vi "DMM Configuration - Update DMM Temp Controls.vi"(8 "error in (no error)":errorcluster, 9 "DMM Temp - Value":T1={"DMM Temp - Transducer Type"=1, "DMM Temp - Thermocouple Type"=6, "DMM Temp - Fixed Reference Junction"=25.0, "DMM Temp - RTD Type"=enum."Pt3851", "DMM Temp - RTD Resistance"=100.0, "DMM Temp - Thermistor Type"=enum."44006", "DMM Temp - RTD A"=0.0039083, "DMM Temp - RTD B"=-5.775e-07, "DMM Temp - RTD C"=-4.183e-12, "DMM Temp - Thermistor A"=0.0010295, "DMM Temp - Thermistor B"=0.0002391, "DMM Temp - Thermistor C"=1.568e-07} {"DMM Temp - Thermistor C" format="%#_13g"; "DMM Temp - Thermistor B" format="%#_13g"; "DMM Temp - Thermistor A" format="%#_13g"; "DMM Temp - RTD Resistance" format="%.2f"; "DMM Temp - Fixed Reference Junction" format="%.2f"; "DMM Temp - Thermocouple Type" items=["B"=1, "E"=4, "J"=6, "K"=7, "N"=8, "R"=9, "S"=10, "T"=11]; "DMM Temp - Transducer Type" items=["Thermocouple"=1, "Thermistor"=2, "2-Wire RTD"=3, "4-Wire RTD"=4]}, 11 "Measurement Controls Refs":T6) -> (0 "error out":errorcluster)   [LabVIEW 2016, in "DMM-SWITCH-ScanList System Explorer.lvlib"]
uses:
  DMM-SWITCH-ScanList System Explorer.lvlib
  <instrlib>/niDMM/nidmm.llb/niDMM Transducer Type.ctl
  <instrlib>/niDMM/nidmm.llb/niDMM Thermistor Type.ctl
  <instrlib>/niDMM/nidmm.llb/niDMM RTD Type.ctl
  <instrlib>/niDMM/nidmm.llb/niDMM Thermocouple Type.ctl
  Configuration Controls/DMM Temp.ctl
panel:
  in  "DMM Temp - Thermocouple Type":T3=6 caption="DMM Temp - Thermocouple Type Value" items=["B"=1, "E"=4, "J"=6, "K"=7, "N"=8, "R"=9, "S"=10, "T"=11]
  in  "DMM Temp - RTD Type":T4=enum."Pt3851" caption="DMM Temp - RTD Type Value"
  in  "DMM Temp - Thermistor Type":T5=enum."44006" caption="DMM Temp - Thermistor Type Value"
  in  "DMM Temp - Transducer Type":T2=1 items=["Thermocouple"=1, "Thermistor"=2, "2-Wire RTD"=3, "4-Wire RTD"=4]
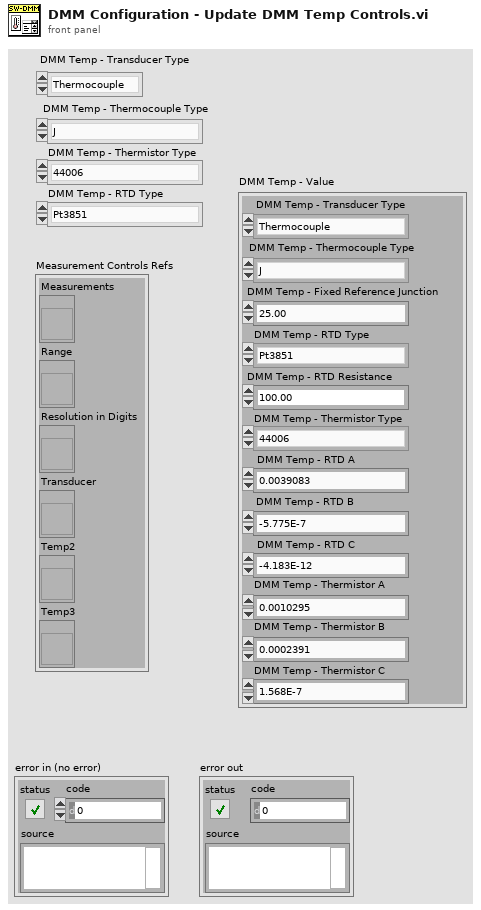
[diagram p1: front panel]
types:
  T1 = typedef "DMM-SWITCH-ScanList System Explorer.lvlib/DMM Temp.ctl" = cluster{"DMM Temp - Transducer Type":T2, "DMM Temp - Thermocouple Type":T3, "DMM Temp - Fixed Reference Junction":dbl, "DMM Temp - RTD Type":T4, "DMM Temp - RTD Resistance":dbl, "DMM Temp - Thermistor Type":T5, "DMM Temp - RTD A":dbl, "DMM Temp - RTD B":dbl, "DMM Temp - RTD C":dbl, "DMM Temp - Thermistor A":dbl, "DMM Temp - Thermistor B":dbl, "DMM Temp - Thermistor C":dbl}
  T2 = typedef "niDMM Transducer Type.ctl" = i32
  T3 = typedef "niDMM Thermocouple Type.ctl" = i32
  T4 = typedef "niDMM RTD Type.ctl" = enum16{"Custom", "Pt3750", "Pt3851", "Pt3911", "Pt3916", "Pt3920", "Pt3928"}
  T5 = typedef "niDMM Thermistor Type.ctl" = enum16{"Custom", "44004", "44006", "44007"}
  T6 = cluster{"Measurements":refnum<vi>, "Range":refnum<vi>, "Resolution in Digits":refnum<vi>, "Transducer":refnum<vi>, "Temp2":refnum<vi>, "Temp3":refnum<vi>}
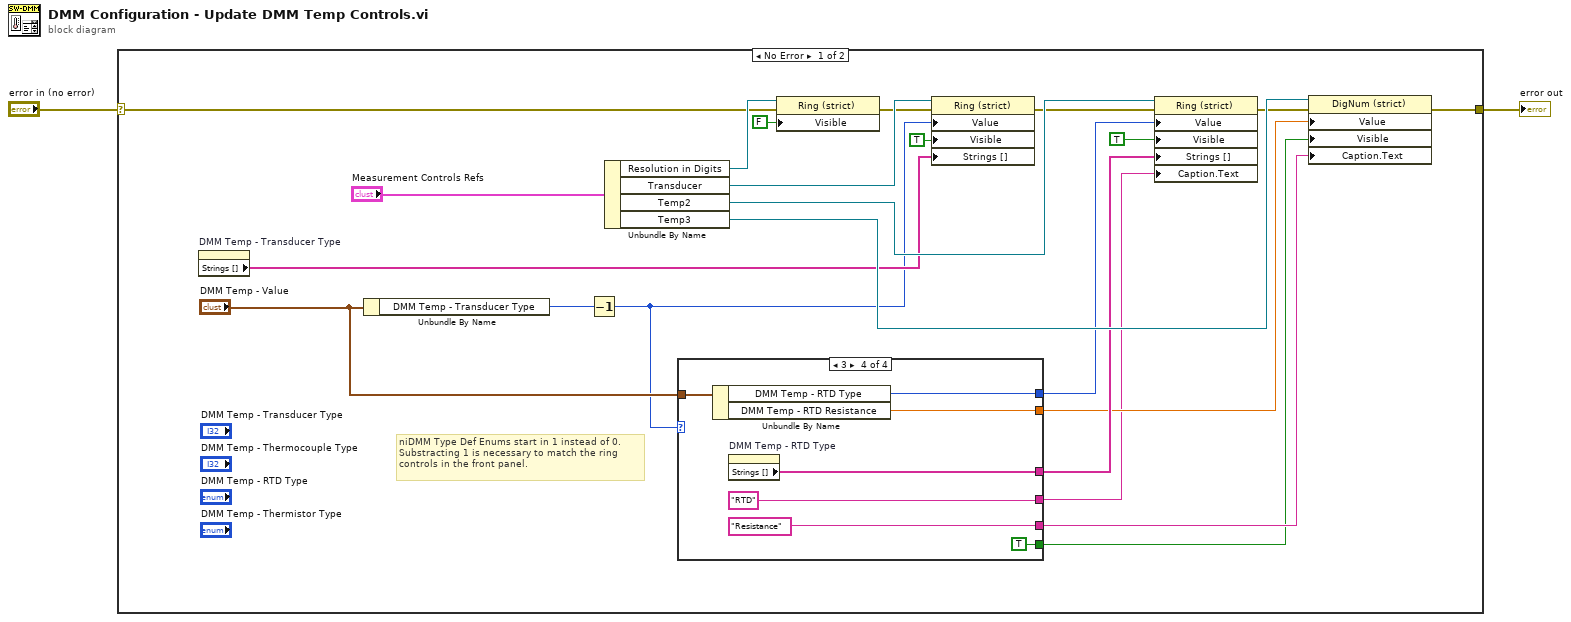
[diagram p0: block diagram]
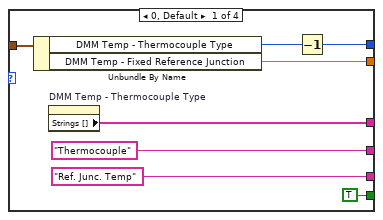
[diagram p2: hidden frame]
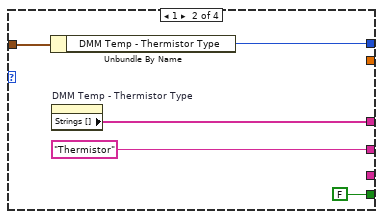
[diagram p3: hidden frame]
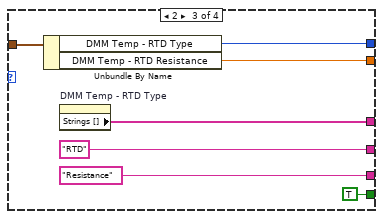
[diagram p4: hidden frame]
diagram:
  n1 = case shown="No Error" "error in (no error)" {
    selector: "error in (no error)" -> [w6 w53]
    tunnel: [w21 w53] -> w2
    frame No Error {
      # "niDMM Type Def Enums start in 1 instead of 0.\nSubstracting 1 is necessary to match the ring \ncontrols in the front panel."
      n2 = property on="DMM Temp - Transducer Type" class="Ring (strict)"() -> ("Strings []"=w20:string[])  [unwired: 2 in, 2 out]
      n3 = Unbundle By Name("DMM Temp - Value") -> ("DMM Temp - Transducer Type"=w5:T2)
      n4 = Decrement(x=w5) -> (x-1=w4:T2)
      n5 = Unbundle By Name("Measurement Controls Refs") -> ("Resolution in Digits"=w25:refnum<vi>, "Transducer"=w24:refnum<vi>, "Temp2"=w23:refnum<vi>, "Temp3"=w22:refnum<vi>)
      n6 = case shown="3" w4 {
        tunnel: "DMM Temp - Value" -> [w33 w38 w45 w52]
        tunnel: [w26 w37 w44 w51] -> w3
        tunnel: [w32 w36 w43 w50] -> w19
        tunnel: [w31 _ w42 w49] -> w17
        tunnel: ["Thermocouple" "Thermistor" "RTD" "RTD"] -> w15
        tunnel: ["Ref. Junc. Temp" _ "Resistance" "Resistance"] -> w14
        tunnel: [TRUE ("Visible") FALSE ("Visible") TRUE ("Visible") TRUE ("Visible")] -> w13
        frame 0, Default {
          n7 = Unbundle By Name(w33) -> ("DMM Temp - Thermocouple Type"=w27:T3, "DMM Temp - Fixed Reference Junction"=w31:dbl)
          n8 = property on="DMM Temp - Thermocouple Type" class="Ring (strict)"() -> ("Strings []"=w32:string[])  [unwired: 2 in, 2 out]
          n9 = Decrement(x=w27) -> (x-1=w26:T3)
        }
        frame 1 {
          n10 = Unbundle By Name(w38) -> ("DMM Temp - Thermistor Type"=w37:T5)
          n11 = property on="DMM Temp - Thermistor Type" class="Enum (strict)"() -> ("Strings []"=w36:string[])  [unwired: 2 in, 2 out]
        }
        frame 2 {
          n12 = Unbundle By Name(w45) -> ("DMM Temp - RTD Type"=w44:T4, "DMM Temp - RTD Resistance"=w42:dbl)
          n13 = property on="DMM Temp - RTD Type" class="Enum (strict)"() -> ("Strings []"=w43:string[])  [unwired: 2 in, 2 out]
        }
        frame 3 {
          n14 = Unbundle By Name(w52) -> ("DMM Temp - RTD Type"=w51:T4, "DMM Temp - RTD Resistance"=w49:dbl)
          n15 = property on="DMM Temp - RTD Type" class="Enum (strict)"() -> ("Strings []"=w50:string[])  [unwired: 2 in, 2 out]
        }
      }
      n16 = property on="Property Node" class="Ring (strict)"(reference=w25, error in=w6, "Visible"=FALSE) -> (error out=w11:errorcluster)  [unwired: 1 out]
      n17 = property on="Property Node" class="Ring (strict)"(reference=w24, error in=w11, "Value"=w4, "Visible"=TRUE, "Strings []"=w20) -> (error out=w9:errorcluster)  [unwired: 1 out]
      n18 = property on="Property Node" class="Ring (strict)"(reference=w23, error in=w9, "Value"=w3, "Visible"=TRUE, "Strings []"=w19, "Caption.Text"=w15) -> (error out=w7:errorcluster)  [unwired: 1 out]
      n19 = property on="Property Node" class="DigNum (strict)"(reference=w22, error in=w7, "Value"=w17, "Visible"=w13, "Caption.Text"=w14) -> (error out=w21:errorcluster)  [unwired: 1 out]
    }
    frame Error {
    }
  }
  "error out" <- w2
